vi "Get Storage Ref.vi"(11 "Init (F)":bool) -> (3 "Storage":refnum<data-value>)   [LabVIEW 2013, in "MQTT Server.lvlib" / "StoredSessions.lvclass"]
uses:
  StoredSessions.lvclass
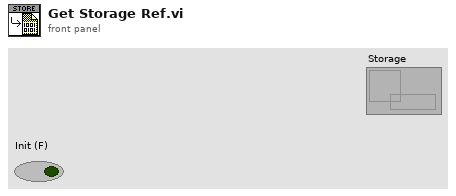
[diagram p1: front panel]
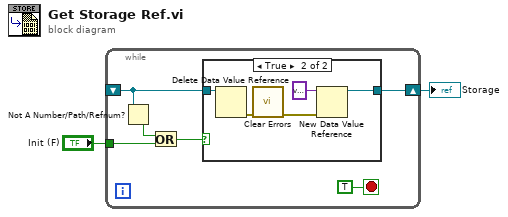
[diagram p0: block diagram]
diagram:
  n1 = while {
    shift-right: [w8] -> w2
    shift-left: _ -> [w6]
    tunnel: "Init (F)" -> [w5]
    stop <- TRUE stop-if-true
    n2 = Not A Number/Path/Refnum?(number/path/refnum=w6) -> (NaN/Path/Refnum?=w4:bool)
    n3 = Or(x=w4, y=w5) -> (x .or. y?=w3:bool)
    n4 = case shown="True" w3 {
      tunnel: [w9 w13] -> w8
      tunnel: w6 -> [w9 w12]
      frame False {
      }
      frame True {
        n5 = Delete Data Value Reference(data value reference=w12) -> (error out=w11:errorcluster)  [unwired: 1 in, 1 out]
        n6 = call <vilib>:"Clear Errors.vi"("error in (no error)"=w11) -> ("error out"=w10:errorcluster)  [unwired: 6 in]
        n7 = New Data Value Reference(data value=variant ("storage"), error in=w10) -> (data value reference=w13:refnum<data-value>)  [unwired: 1 out]
      }
    }
  }
  "Storage" <- w2
